vi "Q8381 REF LEVEL_PEAK.vi"(1 "GPIB Address":u16=8 max=31 step=1, 2 "VISA resource name":refnum<visa-resource-name>) -> (0 "GPIB Status":bool)   [LabVIEW 2017]
panel:
  out "Program Code":string
  # "REF  LEVEL__PEAK"
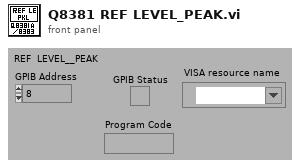
[diagram p1: front panel]
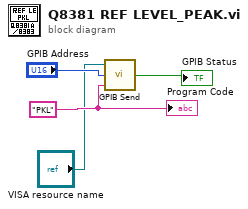
[diagram p0: block diagram]
diagram:
  w2 = "PKL"
  n1 = call "GPIB Send.vi"("Command String"=w2, "Address"="GPIB Address", "VISA resource name"="VISA resource name") -> ("Error"=→"GPIB Status":bool)
  "Program Code" <- w2
